vi "Inst_DAQ.vi"(8 "error in":errorcluster, 10 "All Message Queues in":T1, 11 "Prueba31 in":refnum<class "Prueba21.lvclass">) -> (0 "error out":errorcluster)   [LabVIEW 2019, in "Prueba21.lvclass"]
uses:
  Prueba21.lvclass
  QMH/Message Queue/All Message Queues.ctl
  QMH/Message Queue/Message Cluster.ctl
  Prueba21.lvclass/Prueba21.ctl
  <vilib>/DAQmx/read.llb/DAQmx Read (Analog Wfm 1Chan NSamp).vi
  <vilib>/DAQmx/read.llb/DAQmx Read (Analog Wfm 1Chan 1Samp).vi
  <vilib>/Utility/error.llb/Error Cluster From Error Code.vi
  QMH/Message Queue/Enqueue Message (Single).vi
  <vilib>/DAQmx/miscellaneous.llb/DAQmx Fill In Error Info.vi
  <vilib>/express/express analysis/Spectral/Block/exnSpectralBlock spectral measurements RMS poly.vi
  <vilib>/express/express analysis/Spectral/Block/exnSpectralBlock spectral measurements RMS array WFM.vi
  <vilib>/ErrorRing/Error Ring.xnode
  <vilib>/express/express analysis/Spectral/XNode/ExpressSpectralMeasurementsBlockNode.xnode
  QMH/Message Queue/Message Queue.lvlib
panel:
  out "All States":string[](array[string])
  out "Actual State":string
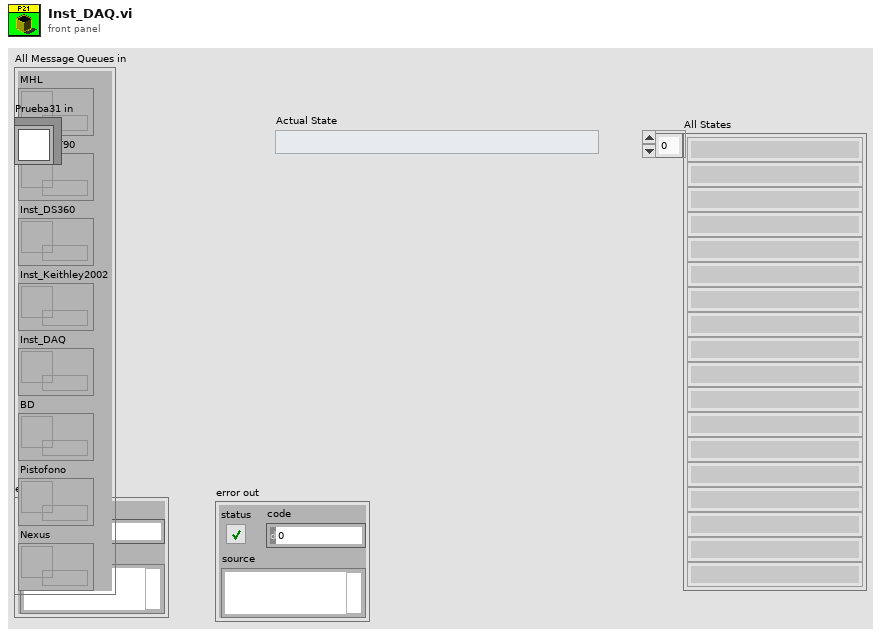
[diagram p1: front panel]
types:
  T1 = typedef "Message Queue.lvlib/All Message Queues.ctl" = cluster{"MHL":refnum<queue>, "Inst_CNT90":refnum<queue>, "Inst_DS360":refnum<queue>, "Inst_Keithley2002":refnum<queue>, "Inst_DAQ":refnum<queue>, "BD":refnum<queue>, "Pistofono":refnum<queue>, "Nexus":refnum<queue>}
  T2 = cluster{"averaging mode":u16, "weighting mode":u16, "number of averages":u32}
  T3 = cluster{"dB On (F)":bool, "unwrap phase (F)":bool, "convert to degree (F)":bool}
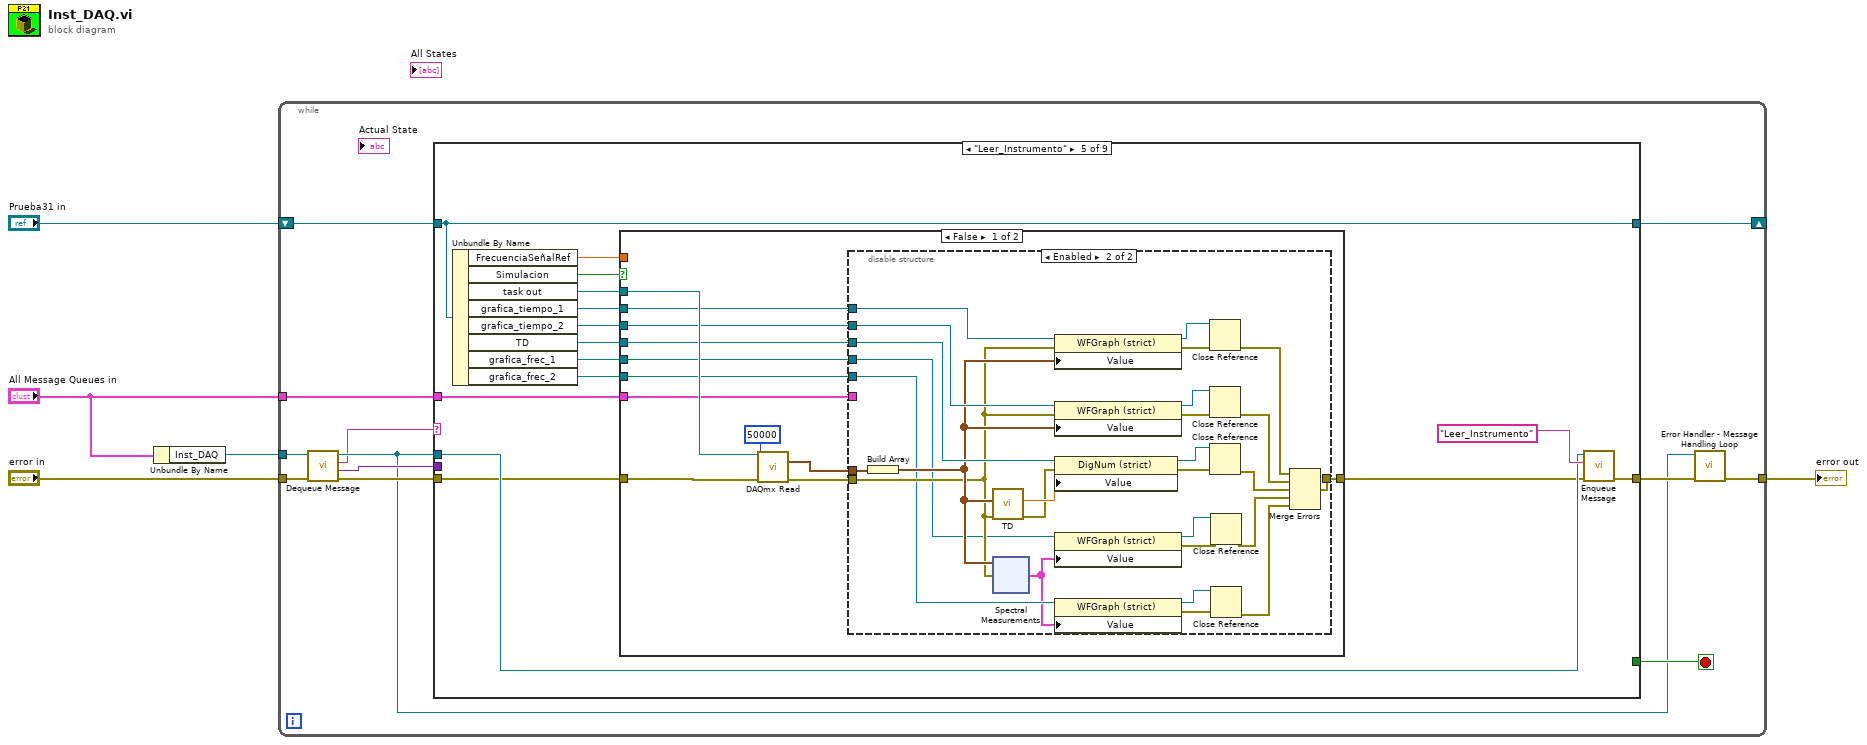
[diagram p0: block diagram]
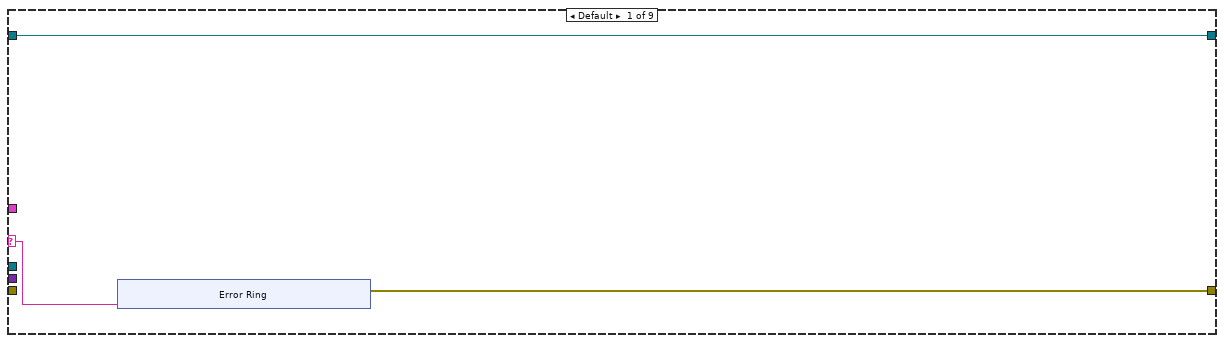
[diagram p2: hidden frame]
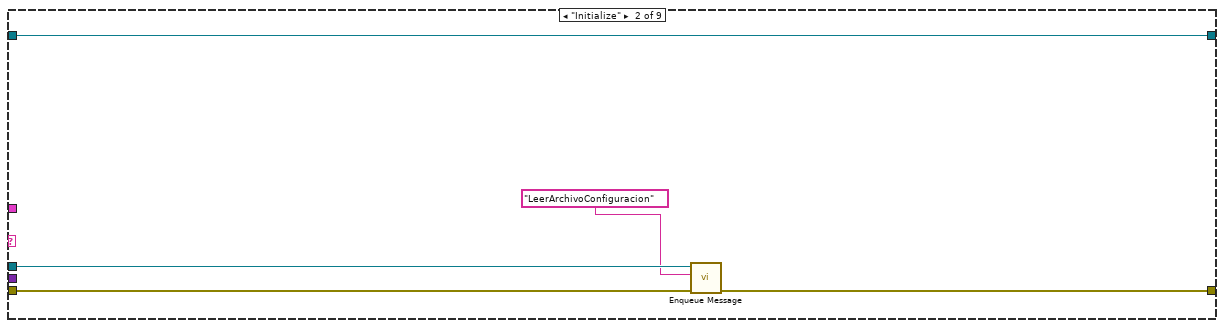
[diagram p3: hidden frame]
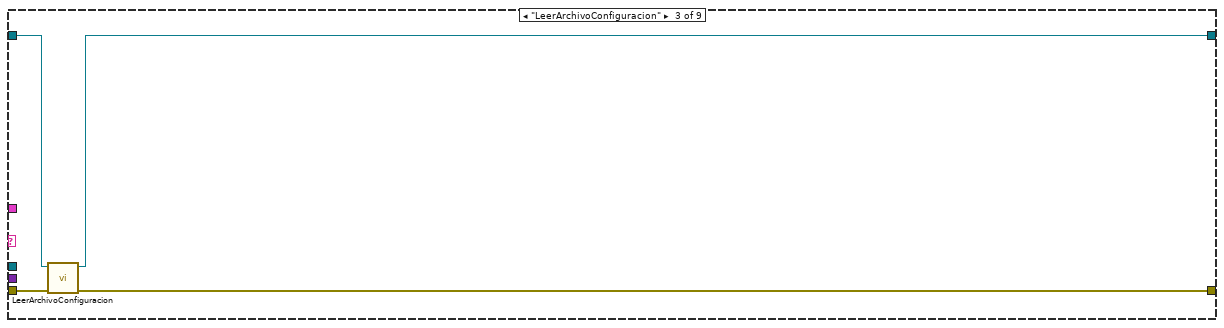
[diagram p4: hidden frame]
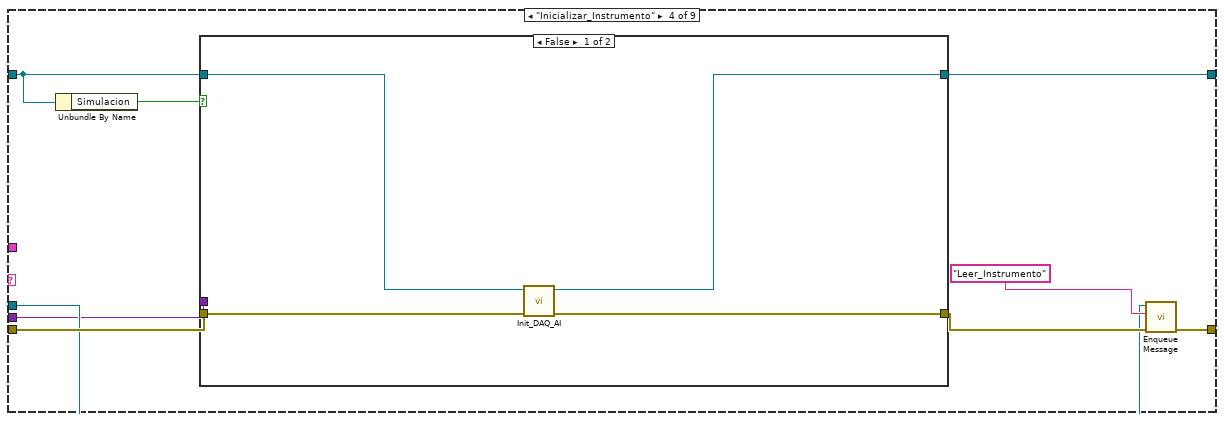
[diagram p5: hidden frame]
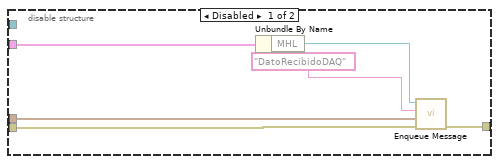
[diagram p7: hidden frame]
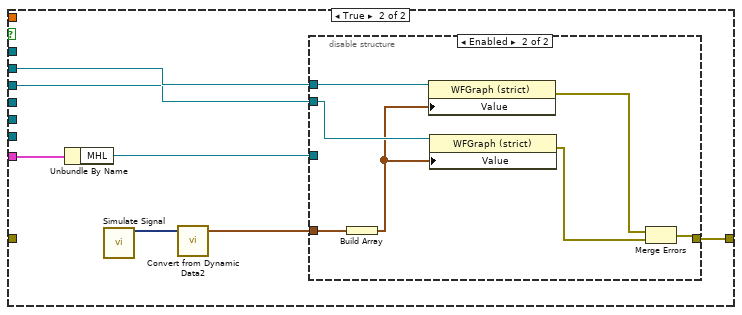
[diagram p8: hidden frame]
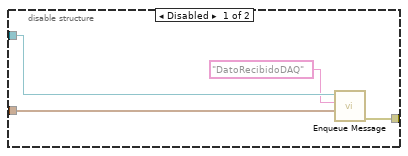
[diagram p9: hidden frame]
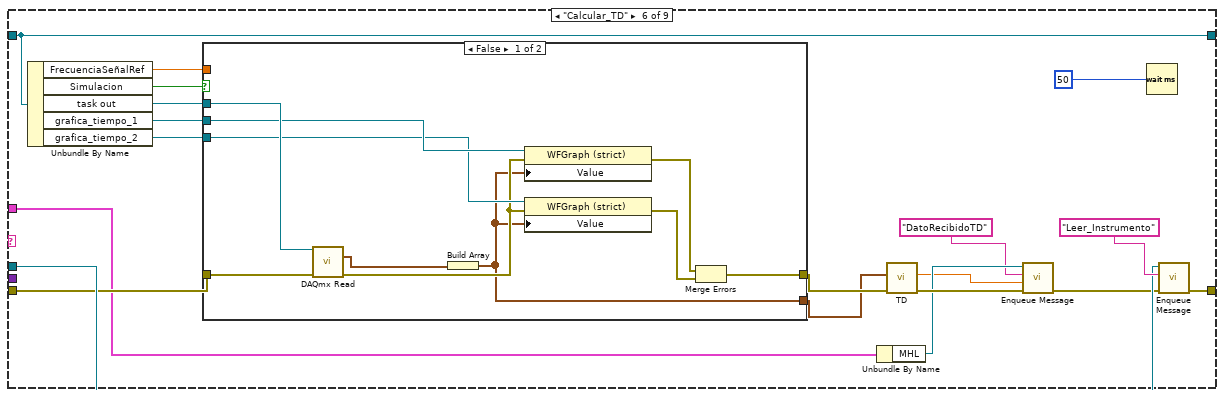
[diagram p10: hidden frame]
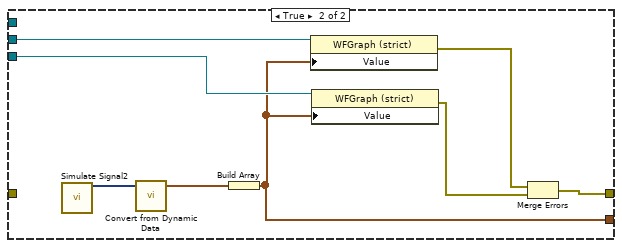
[diagram p11: hidden frame]
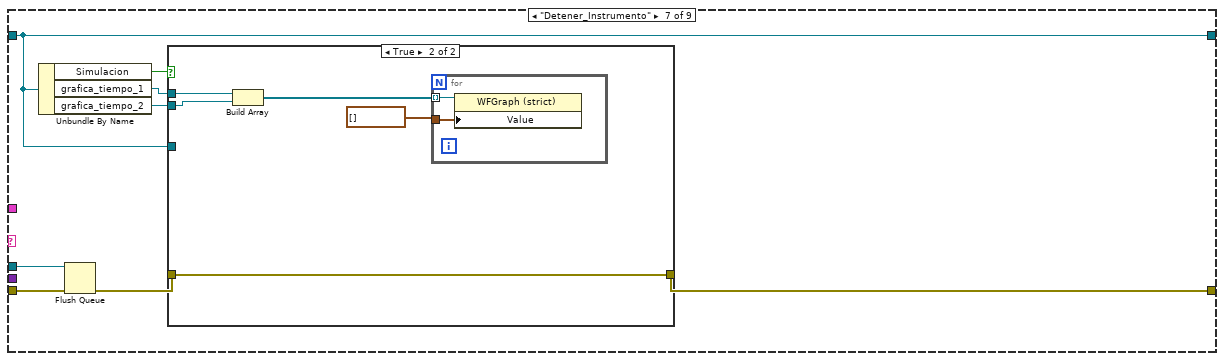
[diagram p12: hidden frame]
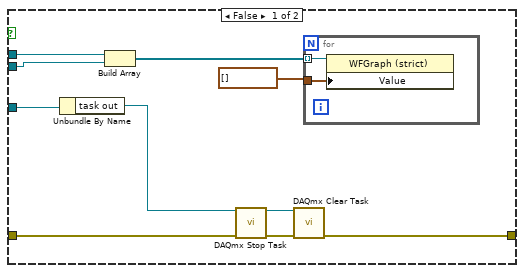
[diagram p13: hidden frame]
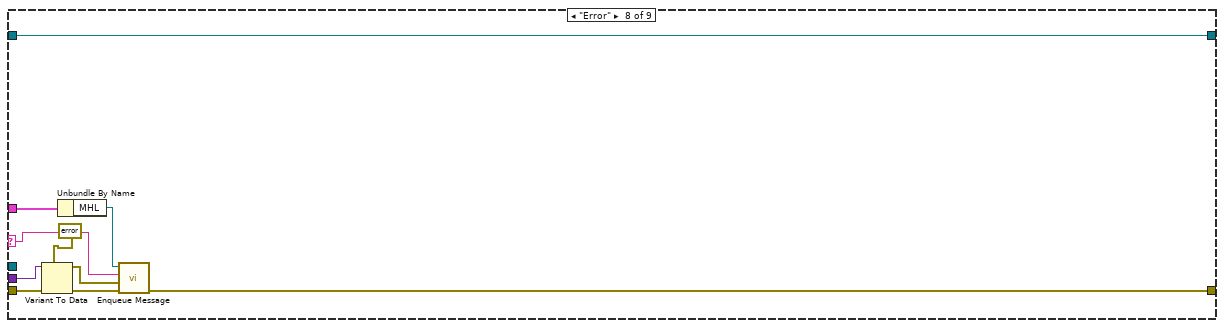
[diagram p14: hidden frame]
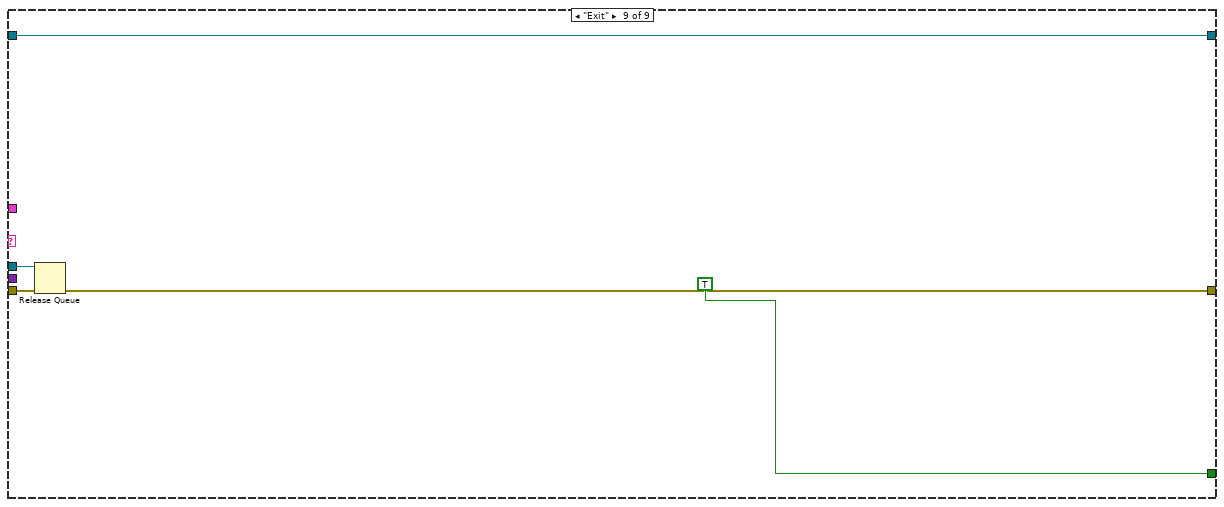
[diagram p15: hidden frame]
diagram:
  n1 = Unbundle By Name("All Message Queues in") -> ("Inst_DAQ"=w3:refnum<queue>)
  n2 = while {
    tunnel: "error in" -> [w17]
    tunnel: w3 -> [w16]
    tunnel: "All Message Queues in" -> [w15]
    tunnel: [w8] -> w1
    shift-right: [w11] -> _
    shift-left: "Prueba31 in" -> [w14]
    stop <- w10 stop-if-true
    n3 = call "Dequeue Message.vi"("error in (no error)"=w17, "Message Queue"=w16) -> ("error out"=w12:errorcluster, "Message Data"=w13:variant, "Message"=w6:string, "dup Message Queue"=w7:refnum<queue>)  [unwired: 6 in]
    n4 = case shown="\"Leer_Instrumento\"" w6 {
      selector: w6 -> [w20 _ _ _ _ _ _ w208 _]
      tunnel: w15 -> [_ _ _ _ w61 w145 _ w207 _]
      tunnel: w14 -> [w18 w32 w34 w38 w62 w153 w180 w205 w215]
      tunnel: w7 -> [_ w29 _ w40 w64 w156 w181 _ w217]
      tunnel: w13 -> [_ _ _ w39 _ _ _ w211 _]
      tunnel: w12 -> [_ w30 w36 w45 w63 w154 w182 w212 w218]
      tunnel: [w19 w31 w33 w42 w65 w157 w184 w204 w214] -> w9
      tunnel: [w18 w32 w35 w37 w62 w153 w180 w205 w215] -> w11
      tunnel: [_ _ _ _ _ _ _ _ TRUE] -> w10
      frame Default {
        n5 = xnode "Error Ring"("parameter 0"=w20) -> ("error out"=w19:errorcluster)
      }
      frame "Initialize" {
        n6 = call-poly "Enqueue Message.vi"("error in (no error)"=w30, "Message"="LeerArchivoConfiguracion", "Message Queue"=w29) -> ("error out"=w31:errorcluster)  [unwired: 7 in, 1 out]
      }
      frame "LeerArchivoConfiguracion" {
        n7 = call "LeerArchivoConfiguracion.vi"("error in"=w36, "Prueba31 in"=w34) -> ("error out"=w33:errorcluster, "Prueba31 out"=w35:refnum<class "Prueba21.lvclass">)  [unwired: 8 in]
      }
      frame "Inicializar_Instrumento" {
        n8 = Unbundle By Name(w38) -> ("Simulacion"=w44:bool)
        n9 = case shown="False" w44 {
          tunnel: [w48 w51] -> w41
          tunnel: w45 -> [w49 w51]
          tunnel: w39 -> [_ _]
          tunnel: w38 -> [w47 w50]
          tunnel: [w46 w50] -> w37
          frame False {
            n10 = call "Init_DAQ_AI.vi"("error in (no error)"=w49, "Prueba21_1 in"=w47) -> ("error out"=w48:errorcluster, "Prueba21_1 out"=w46:refnum<class "Prueba21.lvclass">)  [unwired: 8 in]
          }
          frame True {
            # "Simulacion"
          }
        }
        n11 = call-poly "Enqueue Message.vi"("error in (no error)"=w41, "Message"="Leer_Instrumento", "Message Queue"=w40) -> ("error out"=w42:errorcluster)  [unwired: 7 in, 1 out]
      }
      frame "Leer_Instrumento" {
        n12 = Unbundle By Name(w62) -> ("FrecuenciaSeñalRef"=w60:dbl, "Simulacion"=w59:bool, "task out"=w58:refnum<k21>, "grafica_tiempo_1"=w57:refnum<vi>, "grafica_tiempo_2"=w56:refnum<vi>, "TD"=w55:refnum<vi>, "grafica_frec_1"=w53:refnum<vi>, "grafica_frec_2"=w52:refnum<vi>)
        n13 = case shown="False" w59 {
          tunnel: [w76 w125] -> w54
          tunnel: w63 -> [w78 _]
          tunnel: w61 -> [w75 w128]
          tunnel: w60 -> [_ _]
          tunnel: w58 -> [w77 _]
          tunnel: w57 -> [w72 w127]
          tunnel: w56 -> [w71 w126]
          tunnel: w55 -> [w69 _]
          tunnel: w53 -> [w68 _]
          tunnel: w52 -> [w67 _]
          frame False {
            n14 = call-poly <vilib>:"DAQmx Read.vi"("task/channels in"=w77, "number of samples per channel"=50000, "error in"=w78) -> ("data"=w74:waveform(dbl), "error out"=w73:errorcluster)  [unwired: 10 in, 1 out]
            n15 = disable-structure shown="Enabled" {
              disable-tunnel: [w81 w108] -> w76
              disable-tunnel: w75 -> [w84 _]
              disable-tunnel: w74 -> [w83 w111]
              disable-tunnel: w73 -> [w82 w88]
              disable-tunnel: w72 -> [_ w110]
              disable-tunnel: w71 -> [_ w109]
              disable-tunnel: w69 -> [_ w107]
              disable-tunnel: w68 -> [_ w87]
              disable-tunnel: w67 -> [_ w86]
              frame Disabled {
                n16 = Unbundle By Name(w84) -> ("MHL"=w80:refnum<queue>)
                n17 = call-poly "Enqueue Message.vi"("error in (no error)"=w82, "Message Data"=w83, "Message"="DatoRecibidoDAQ", "Message Queue"=w80) -> ("error out"=w81:errorcluster)  [unwired: 6 in, 1 out]
              }
              frame Enabled {
                n18 = Build Array(w111) -> (w89:waveform(dbl)[])
                n19 = call "TD.vi"("error in (no error)"=w88, "Sine"=w89) -> ("error out"=w96:errorcluster, "TD (%)"=w106:dbl)  [unwired: 8 in]
                n20 = xnode ("Spectral Measurements")("Signals"=w89, "error in (no error)"=w88) -> ("FFT - (RMS)"=w85:cluster{"f0":dbl, "df":dbl, "magnitude":dbl[]}[])  [unwired: 2 out]
                n21 = property class="WFGraph (strict)"(reference=w110, error in=w88, "Value"=w89) -> (reference out=w102:refnum<vi>, error out=w103:errorcluster)
                n22 = property class="WFGraph (strict)"(reference=w109, error in=w88, "Value"=w89) -> (reference out=w100:refnum<vi>, error out=w99:errorcluster)
                n23 = property class="DigNum (strict)"(reference=w107, error in=w96, "Value"=w106) -> (reference out=w104:refnum<vi>, error out=w105:errorcluster)
                n24 = property class="WFGraph (strict)"(reference=w87, "Value"=w85) -> (reference out=w93:refnum<vi>, error out=w95:errorcluster)  [unwired: 1 in]
                n25 = property class="WFGraph (strict)"(reference=w86, "Value"=w85) -> (reference out=w92:refnum<vi>, error out=w94:errorcluster)  [unwired: 1 in]
                n26 = Close Reference(reference=w102, error in (no error)=w103) -> (error out=w101:errorcluster)
                n27 = Close Reference(reference=w100, error in (no error)=w99) -> (error out=w98:errorcluster)
                n28 = Close Reference(reference=w104, error in (no error)=w105) -> (error out=w97:errorcluster)
                n29 = Close Reference(reference=w93, error in (no error)=w95) -> (error out=w91:errorcluster)
                n30 = Close Reference(reference=w92, error in (no error)=w94) -> (error out=w90:errorcluster)
                n31 = Merge Errors(w101, w98, w97, w91, w90) -> (w108:errorcluster)
              }
            }
          }
          frame True {
            n32 = Unbundle By Name(w128) -> ("MHL"=w124:refnum<queue>)
            n33 = call "Simulate Signal"() -> ("Sine"=w122:dynamicdata)  [unwired: 14 in, 1 out]
            n34 = call "Convert from Dynamic Data2"("Dynamic Data Type"=w122) -> ("Waveform"=w123:waveform(dbl))  [unwired: 3 in]
            n35 = disable-structure shown="Enabled" {
              disable-tunnel: [w131 w137] -> w125
              disable-tunnel: w124 -> [w130 _]
              disable-tunnel: w123 -> [w132 w134]
              disable-tunnel: w127 -> [_ w139]
              disable-tunnel: w126 -> [_ w138]
              frame Disabled {
                n36 = call-poly "Enqueue Message.vi"("Message Data"=w132, "Message"="DatoRecibidoDAQ", "Message Queue"=w130) -> ("error out"=w131:errorcluster)  [unwired: 7 in, 1 out]
              }
              frame Enabled {
                n37 = Build Array(w134) -> (w135:waveform(dbl)[])
                n38 = property class="WFGraph (strict)"(reference=w139, "Value"=w135) -> (error out=w133:errorcluster)  [unwired: 1 in, 1 out]
                n39 = property class="WFGraph (strict)"(reference=w138, "Value"=w135) -> (error out=w136:errorcluster)  [unwired: 1 in, 1 out]
                n40 = Merge Errors(w133, w136) -> (w137:errorcluster)
              }
            }
          }
        }
        n41 = call-poly "Enqueue Message.vi"("error in (no error)"=w54, "Message"="Leer_Instrumento", "Message Queue"=w64) -> ("error out"=w65:errorcluster)  [unwired: 7 in, 1 out]
      }
      frame "Calcular_TD" {
        n42 = Unbundle By Name(w153) -> ("FrecuenciaSeñalRef"=w152:dbl, "Simulacion"=w151:bool, "task out"=w150:refnum<k21>, "grafica_tiempo_1"=w149:refnum<vi>, "grafica_tiempo_2"=w148:refnum<vi>)
        n43 = case shown="False" w151 {
          tunnel: [w166 w174] -> w147
          tunnel: w154 -> [w168 _]
          tunnel: w152 -> [_ _]
          tunnel: w150 -> [w167 _]
          tunnel: w149 -> [w164 w176]
          tunnel: w148 -> [w163 w175]
          tunnel: [w159 w169] -> w144
          frame False {
            n44 = call-poly <vilib>:"DAQmx Read.vi"("task/channels in"=w167, "error in"=w168) -> ("data"=w165:waveform(dbl), "error out"=w160:errorcluster)  [unwired: 11 in, 1 out]
            n45 = Build Array(w165) -> (w159:waveform(dbl)[])
            n46 = property class="WFGraph (strict)"(reference=w164, error in=w160, "Value"=w159) -> (error out=w162:errorcluster)  [unwired: 1 out]
            n47 = property class="WFGraph (strict)"(reference=w163, error in=w160, "Value"=w159) -> (error out=w161:errorcluster)  [unwired: 1 out]
            n48 = Merge Errors(w162, w161) -> (w166:errorcluster)
          }
          frame True {
            n49 = call "Simulate Signal2"() -> ("Sine"=w172:dynamicdata)  [unwired: 14 in, 1 out]
            n50 = call "Convert from Dynamic Data"("Dynamic Data Type"=w172) -> ("Waveform"=w173:waveform(dbl))  [unwired: 3 in]
            n51 = Build Array(w173) -> (w169:waveform(dbl)[])
            n52 = property class="WFGraph (strict)"(reference=w176, "Value"=w169) -> (error out=w170:errorcluster)  [unwired: 1 in, 1 out]
            n53 = property class="WFGraph (strict)"(reference=w175, "Value"=w169) -> (error out=w171:errorcluster)  [unwired: 1 in, 1 out]
            n54 = Merge Errors(w170, w171) -> (w174:errorcluster)
          }
        }
        n55 = Unbundle By Name(w145) -> ("MHL"=w142:refnum<queue>)
        n56 = call "TD.vi"("error in (no error)"=w147, "Sine"=w144) -> ("error out"=w146:errorcluster, "TD (%)"=w140:dbl)  [unwired: 8 in]
        n57 = call-poly "Enqueue Message.vi"("error in (no error)"=w146, "Message Data"=w140, "Message"="DatoRecibidoTD", "Message Queue"=w142) -> ("error out"=w143:errorcluster)  [unwired: 6 in, 1 out]
        n58 = Wait (ms)(milliseconds to wait=u32 50) -> ()  [unwired: 1 out]
        n59 = call-poly "Enqueue Message.vi"("error in (no error)"=w143, "Message"="Leer_Instrumento", "Message Queue"=w156) -> ("error out"=w157:errorcluster)  [unwired: 7 in, 1 out]
      }
      frame "Detener_Instrumento" {
        n60 = Unbundle By Name(w180) -> ("Simulacion"=w179:bool, "grafica_tiempo_1"=w178:refnum<vi>, "grafica_tiempo_2"=w177:refnum<vi>)
        n61 = Flush Queue(queue=w181, error in (no error)=w182) -> (error out=w183:errorcluster)  [unwired: 2 out]
        n62 = case shown="True" w179 {
          tunnel: [w191 w201] -> w184
          tunnel: w183 -> [w192 w201]
          tunnel: w180 -> [w190 _]
          tunnel: w177 -> [w187 w200]
          tunnel: w178 -> [w186 w199]
          frame False {
            n63 = Unbundle By Name(w190) -> ("task out"=w189:refnum<k21>)
            n64 = Build Array(w186, w187) -> (w188:refnum<vi>[])
            n65 = call <vilib>:"DAQmx Stop Task.vi"("task/channels in"=w189, "error in"=w192) -> ("task out"=w193:refnum<k21>, "error out"=w194:errorcluster)  [unwired: 12 in]
            n66 = call <vilib>:"DAQmx Clear Task.vi"("task in"=w193, "error in"=w194) -> ("error out"=w191:errorcluster)  [unwired: 13 in]
            n67 = for {
              tunnel: w188 -> [w196] mode=indexing
              tunnel: waveform(dbl)[] [] ("grafica_tiempo_2") -> [w195]
              n68 = property on="Property Node" class="WFGraph (strict)"(reference=w196, "Value"=w195) -> ()  [unwired: 1 in, 2 out]
            }
          }
          frame True {
            n69 = Build Array(w199, w200) -> (w198:refnum<vi>[])
            n70 = for {
              tunnel: w198 -> [w203] mode=indexing
              tunnel: waveform(dbl)[] [] ("grafica_tiempo_2") -> [w202]
              n71 = property on="Property Node" class="WFGraph (strict)"(reference=w203, "Value"=w202) -> ()  [unwired: 1 in, 2 out]
            }
          }
        }
      }
      frame "Error" {
        n72 = Variant To Data(error in=w212, type=errorcluster {"status"=FALSE, "code"=0, "source"=""} ("error constant"), Variant=w211) -> (data=w209:errorcluster, error out=w210:errorcluster)
        n73 = Unbundle By Name(w207) -> ("MHL"=w206:refnum<queue>)
        n74 = call-poly "Enqueue Message.vi"("error in (no error)"=w210, "Message Data"=w209, "Message"=w208, "Message Queue"=w206) -> ("error out"=w204:errorcluster)  [unwired: 6 in, 1 out]
      }
      frame "Exit" {
        n75 = Release Queue(queue=w217, error in (no error)=w218) -> (error out=w214:errorcluster)  [unwired: 1 in, 2 out]
      }
    }
    n76 = call "Error Handler - Message Handling Loop.vi"("error in (no error)"=w9, "Message Queue"=w7) -> ("dup error in"=w8:errorcluster)  [unwired: 8 in, 1 out]
  }
  "error out" <- w1
